vi "Finalize Settings 1.0.vi"(8 "error in (no error)":errorcluster, 11 "configuration 1.0":T1) -> (0 "error out":errorcluster, 2 "settings version":T2, 3 "settings 1.0":cluster{"key":string, "value":string}[](array[cluster]))   [LabVIEW 2017, in "DSF Core.lvlib" / "Plugin Configuration.lvclass"]
uses:
  Plugin Configuration.lvclass
  Typedefs/DSF Version Info.ctl
  DSF Core.lvlib
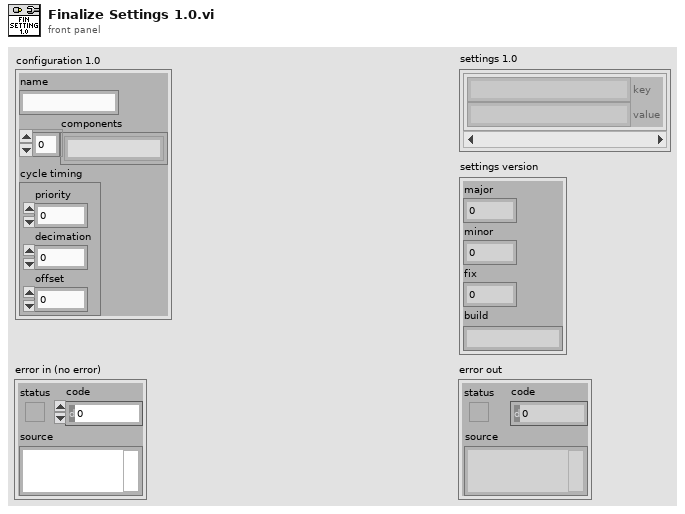
[diagram p1: front panel]
types:
  T1 = cluster{"name":string, "components":string[], "cycle timing":cluster{"priority":u64, "decimation":u64, "offset":u64}}
  T2 = typedef "DSF Core.lvlib/DSF Version Info.ctl" = cluster{"major":u32, "minor":u32, "fix":u32, "build":string}
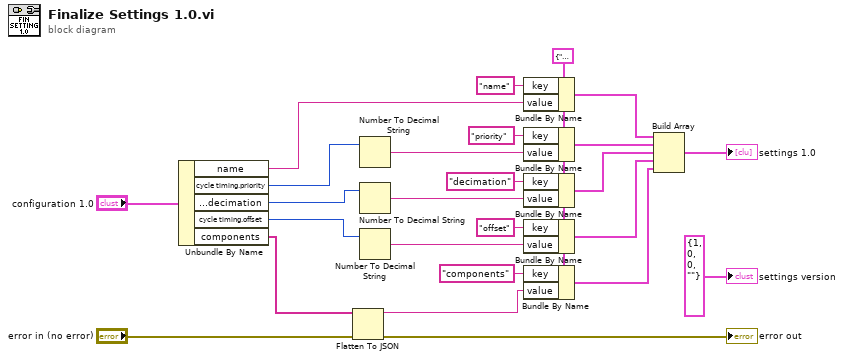
[diagram p0: block diagram]
diagram:
  w3 = cluster{"key":string, "value":string} {"key"="", "value"=""} ("setting")
  n1 = Unbundle By Name("configuration 1.0") -> ("name"=w18:string, "cycle timing.priority"=w14:u64, "cycle timing.decimation"=w13:u64, "cycle timing.offset"=w12:u64, "components"=w5:string[])
  n2 = Flatten To JSON(anything=w5, error in (no error)="error in (no error)") -> (JSON string=w2:string, 11:→"error out":errorcluster)  [unwired: 1 in]
  n3 = Number To Decimal String(number=w14) -> (decimal integer string=w17:string)  [unwired: 1 in]
  n4 = Number To Decimal String(number=w13) -> (decimal integer string=w16:string)  [unwired: 1 in]
  n5 = Number To Decimal String(number=w12) -> (decimal integer string=w15:string)  [unwired: 1 in]
  n6 = Bundle By Name(cluster=w3, "key"="name", "value"=w18) -> (w25:cluster{"key":string, "value":string})
  n7 = Bundle By Name(cluster=w3, "key"="priority", "value"=w17) -> (w24:cluster{"key":string, "value":string})
  n8 = Bundle By Name(cluster=w3, "key"="decimation", "value"=w16) -> (w23:cluster{"key":string, "value":string})
  n9 = Bundle By Name(cluster=w3, "key"="offset", "value"=w15) -> (w11:cluster{"key":string, "value":string})
  n10 = Bundle By Name(cluster=w3, "key"="components", "value"=w2) -> (w1:cluster{"key":string, "value":string})
  n11 = Build Array(w25, w24, w23, w11, w1) -> (→"settings 1.0":cluster{"key":string, "value":string}[])
  "settings version" <- T2 {"major"=1, "minor"=0, "fix"=0, "build"=""} ("settings version")
